vi "Run Protocol.vi"(8 "error in (no error)":errorcluster, 11 "Time Protocol in":refnum<class "Time Protocol.lvclass">) -> (0 "error out":errorcluster, 3 "Time Protocol out":refnum<class "Time Protocol.lvclass">)   [LabVIEW 2013, in "Time Protocol Actor.lvlib" / "Time Protocol.lvclass"]
uses:
  Time Protocol.lvclass
  Time Protocol.lvclass/Time Protocol.ctl
  Read History.vi
  Read Code.vi
  Read State.vi
  PluginInterface/PluginInterface.lvlibp/PluginInterfaceClass/Read DVR.vi
  <vilib>/Utility/file.llb/Read From Spreadsheet File (string).vi
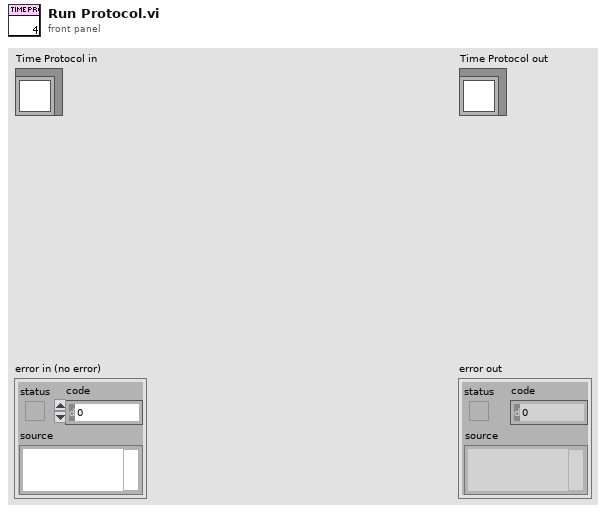
[diagram p1: front panel]
types:
  T1 = enum32{"Pause Button", "Play Button", "Media Stop Button"}
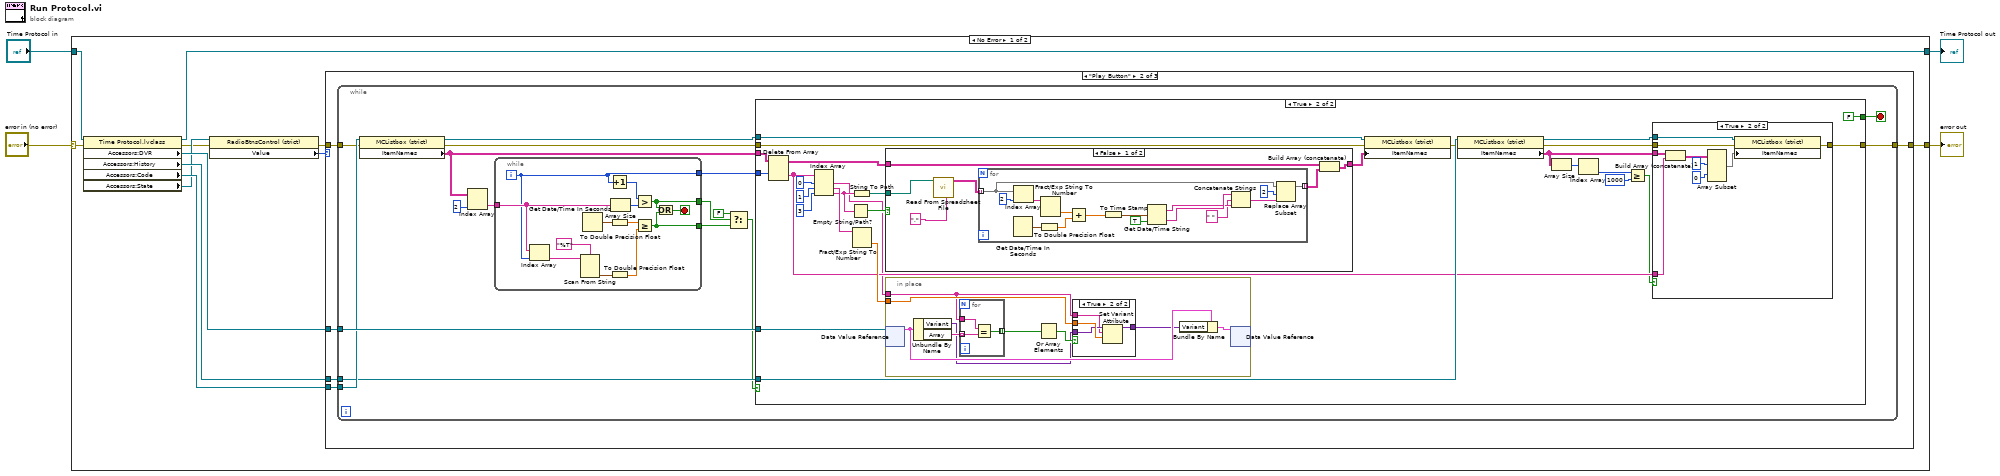
[diagram p0: block diagram]
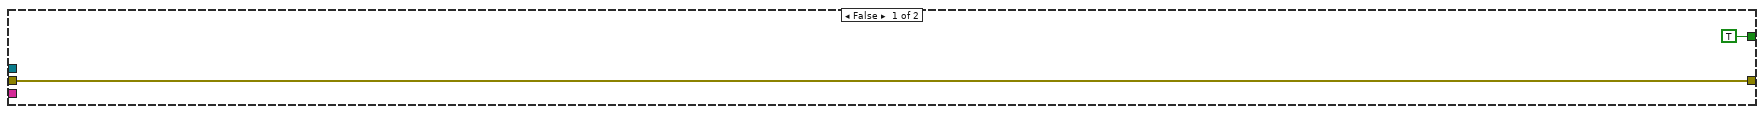
[diagram p3: hidden frame]
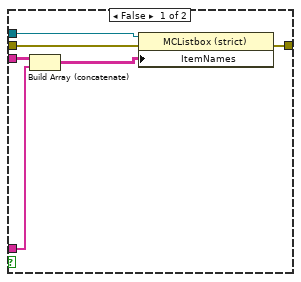
[diagram p5: hidden frame]
diagram:
  n1 = case shown="No Error" "error in (no error)" {
    selector: "error in (no error)" -> [w6 w137]
    tunnel: [w5 w137] -> w3
    tunnel: [w13 w136] -> w1
    tunnel: "Time Protocol in" -> [w12 w136]
    frame No Error {
      n2 = property class="Time Protocol.lvclass"(reference=w12, error in=w6) -> (reference out=w13:refnum<class "Time Protocol.lvclass">, error out=w7:errorcluster, "Accessors:DVR"=w11:refnum<data-value>, "Accessors:History"=w10:refnum<vi>, "Accessors:Code"=w9:refnum<vi>, "Accessors:State"=w8:refnum<vi>)
      n3 = property class="RadioBtnsControl (strict)"(reference=w8, error in=w7) -> (error out=w15:errorcluster, "Value"=w14:T1)  [unwired: 1 out]
      n4 = case shown="\"Play Button\"" w14 {
        tunnel: w11 -> [_ w21 _]
        tunnel: [w16 w18 w135] -> w5
        tunnel: w9 -> [_ w20 _]
        tunnel: w15 -> [w16 w19 w135]
        tunnel: w10 -> [_ w17 _]
        frame "Pause Button", Default {
        }
        frame "Play Button" {
          n5 = while {
            tunnel: w21 -> [w37]
            tunnel: w20 -> [w36]
            tunnel: w19 -> [w35]
            tunnel: [w29] -> w18
            tunnel: w17 -> [w27]
            stop <- w26 stop-if-true
            n6 = property class="MCListbox (strict)"(reference=w36, error in=w35) -> (reference out=w30:refnum<vi>, error out=w31:errorcluster, "ItemNames"=w32:string[][])
            n7 = Index Array(array=w32, index (col)=2 ("disabled index (col)")) -> (element=w33:string[])  [unwired: 1 in]
            n8 = while {
              tunnel: w33 -> [w127]
              tunnel: [w124] -> w28
              tunnel: [w123] -> w24
              tunnel: [w122] -> w25
              i -> [w124]
              stop <- w125 stop-if-true
              n9 = Index Array(array=w127, index=w124) -> (element=w126:string)
              n10 = Scan From String(format string="%T", input string=w126) -> (output 1=w133:timestamp)  [unwired: 3 in, 3 out]
              n11 = Get Date/Time In Seconds() -> (seconds since 1Jan1904=w132:timestamp)
              n12 = Increment(x=w124) -> (x+1=w129:i32)
              n13 = To Double Precision Float(number=w132) -> (double precision float=w130:dbl)
              n14 = To Double Precision Float(number=w133) -> (double precision float=w131:dbl)
              n15 = Array Size(array=w127) -> (size(s)=w128:i32)
              n16 = Greater?(x=w129, y=w128) -> (0:w122:bool)
              n17 = Greater Or Equal?(x=w130, y=w131) -> (x >= y?=w123:bool)
              n18 = Or(x=w122, y=w123) -> (x .or. y?=w125:bool)
            }
            n19 = Select(t=FALSE, s=w25, f=w24) -> (s? t:f=w23:bool)
            n20 = case shown="True" w23 {
              tunnel: w37 -> [_ w67]
              tunnel: w32 -> [_ w66]
              tunnel: w31 -> [w39 w54]
              tunnel: w30 -> [_ w60]
              tunnel: [w39 w41] -> w29
              tunnel: w28 -> [_ w59]
              tunnel: w27 -> [_ w56]
              tunnel: [TRUE FALSE] -> w26
              frame False {
              }
              frame True {
                n21 = Delete From Array(array=w66, index (row)=w59) -> (deleted portion=w53:string[], array with subset deleted=w48:string[][])  [unwired: 2 in]
                n22 = Index Array(array=w53, index #1=0 ("index"), index #2=1 ("index"), index #3=3 ("index")) -> (element #1=w40:string, element #2=w62:string, element #3=w50:string)
                n23 = Empty String/Path?(string/path=w50) -> (empty?=w51:bool)
                n24 = String To Path(string=w50) -> (path=w49:path)
                n25 = Fract/Exp String To Number(string=w62) -> (number=w61:dbl)  [unwired: 3 in, 1 out]
                n26 = case shown="False" w51 {
                  tunnel: w49 -> [w105 _]
                  tunnel: w48 -> [w103 w121]
                  tunnel: [w101 w121] -> w47
                  frame False {
                    n27 = call-poly <vilib>:"Read From Spreadsheet File.vi"("delimiter (\\t)"="," ("delimiter (\\t)"), "file path (dialog if empty)"=w105) -> ("all rows"=w104:string[][])  [unwired: 5 in, 4 out]
                    n28 = for {
                      tunnel: w104 -> [w115] mode=indexing
                      tunnel: [w112] -> w102 mode=indexing
                      n29 = Get Date/Time In Seconds() -> (seconds since 1Jan1904=w119:timestamp)
                      n30 = Index Array(array=w115, index=2) -> (element=w118:string)
                      n31 = To Double Precision Float(number=w119) -> (double precision float=w116:dbl)
                      n32 = Fract/Exp String To Number(string=w118) -> (number=w117:dbl)  [unwired: 3 in, 1 out]
                      n33 = Add(x=w117, y=w116) -> (x+y=w113:dbl)
                      n34 = To Time Stamp(1:w113) -> (0:w108:timestamp)
                      n35 = Get Date/Time String(seconds (now)=w108, want seconds? (F)=TRUE) -> (date string=w110:string, time string=w111:string)  [unwired: 1 in]
                      n36 = Concatenate Strings(w111, " " ("string"), w110) -> (w107:string)
                      n37 = Replace Array Subset(array=w115, new element=w107, index=2) -> (w112:string[])
                    }
                    n38 = Build Array (concatenate)(w103, w102) -> (w101:string[][])
                  }
                  frame True {
                  }
                }
                n39 = in-place {
                  in-place-border: w61 -> [w71]
                  in-place-border: w40 -> [w69]
                  n40 = in-place-dvr #1(w67) -> (w75:cluster{"Array":string[], "Variant":variant})  [unwired: 1 out]
                  n41 = Unbundle By Name(w75) -> ("Variant"=w70:variant, "Array"=w74:string[])
                  n42 = for {
                    tunnel: w74 -> [w84] mode=indexing
                    tunnel: w69 -> [w83]
                    tunnel: [w82] -> w73 mode=indexing
                    n43 = Equal?(x=w83, y=w84) -> (x = y?=w82:bool)
                  }
                  n44 = Or Array Elements(Boolean array=w73) -> (logical OR=w72:bool)
                  n45 = case shown="True" w72 {
                    tunnel: w71 -> [_ w81]
                    tunnel: w70 -> [w77 w80]
                    tunnel: w69 -> [_ w79]
                    tunnel: [w77 w78] -> w68
                    frame False {
                    }
                    frame True {
                      n46 = Set Variant Attribute(Variant=w80, name=w79, value=w81) -> (Variant out=w78:variant)  [unwired: 1 in, 2 out]
                    }
                  }
                  n47 = Bundle By Name(cluster=w75, "Variant"=w68) -> (w76:cluster{"Array":string[], "Variant":variant})
                  n48 = in-place-dvr #1(w76) -> ()  [unwired: 2 out]
                }
                n49 = property class="MCListbox (strict)"(reference=w60, error in=w54, "ItemNames"=w47) -> (error out=w55:errorcluster)  [unwired: 1 out]
                n50 = property class="MCListbox (strict)"(reference=w56, error in=w55) -> (reference out=w57:refnum<vi>, error out=w58:errorcluster, "ItemNames"=w46:string[][])
                n51 = Array Size(array=w46) -> (size(s)=w45:i32[])
                n52 = Index Array(array=w45) -> (element=w44:i32)  [unwired: 1 in]
                n53 = Greater Or Equal?(x=w44, y=1000) -> (x >= y?=w42:bool)
                n54 = case shown="True" w42 {
                  tunnel: w58 -> [w90 w99]
                  tunnel: w57 -> [w89 w98]
                  tunnel: [w88 w97] -> w41
                  tunnel: w46 -> [w87 w96]
                  tunnel: w53 -> [w86 w95]
                  frame False {
                    n55 = Build Array (concatenate)(w87, w86) -> (w85:string[][])
                    n56 = property class="MCListbox (strict)"(reference=w89, error in=w90, "ItemNames"=w85) -> (error out=w88:errorcluster)  [unwired: 1 out]
                  }
                  frame True {
                    n57 = Build Array (concatenate)(w96, w95) -> (w94:string[][])
                    n58 = Array Subset(array=w94, index (row)=1 ("index"), index (col)=0 ("index")) -> (w91:string[][])  [unwired: 2 in]
                    n59 = property class="MCListbox (strict)"(reference=w98, error in=w99, "ItemNames"=w91) -> (error out=w97:errorcluster)  [unwired: 1 out]
                  }
                }
              }
            }
          }
        }
        frame "Media Stop Button" {
        }
      }
    }
    frame Error {
    }
  }
  "error out" <- w3
  "Time Protocol out" <- w1
